vi "Test Compare Clusters.vi"(11 "Dummy In":refnum<class "Example Test Case.lvclass">) -> (0 "error out":errorcluster, 3 "Dummy Out":refnum<class "Example Test Case.lvclass">)   [LabVIEW 2020, in "Example Test Case.lvclass"]
doc: "Test case with comparison"
uses:
  Example Test Case.lvclass
  C:/git/astemes-lunit/source/LUnit Test Case.lvclass
  LUnit Test Case.lvclass/LUnit Test Case.ctl
  c67ca9b7-f05b-4050-9a64-1f171d30ec2c.vi
  Core/LUnit Test Case/Private/Append Pass Result.vi
  Core/LUnit Test Case/Private/Append Fail Result.vi
  c67ca9b7-f05b-4050-9a64-1f171d30ec2c.vi/9c5d11cd-9439-4240-a1ee-d9baace9c924.vi
  Core/LUnit Test Case/Private/Run In UI.vi
  <vilib>/Utility/error.llb/Clear Errors.vi
  Example Test Case.lvclass/Example Test Case.ctl
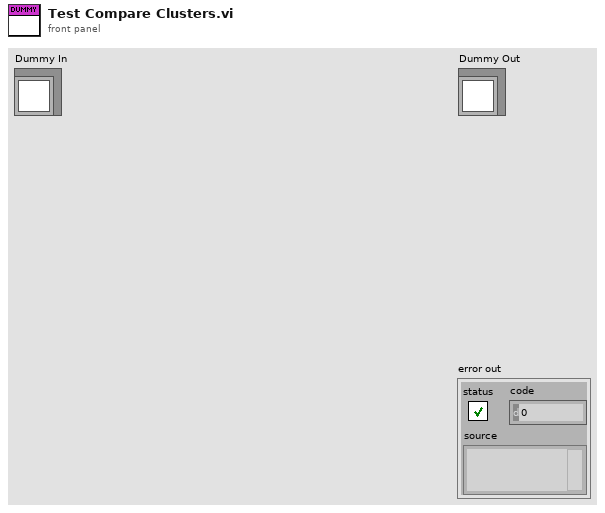
[diagram p1: front panel]
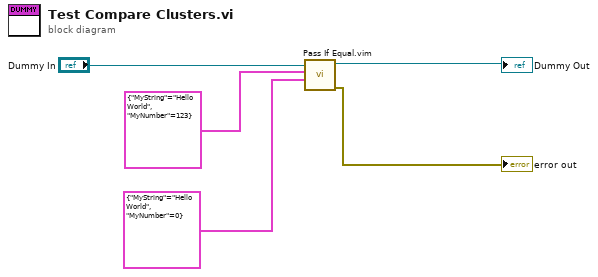
[diagram p0: block diagram]
diagram:
  n1 = call "Pass If Equal.vim"("Actual"=cluster{"MyString":string, "MyNumber":i32} {"MyString"="Hello World", "MyNumber"=0}, "Expected"=cluster{"MyString":string, "MyNumber":i32} {"MyString"="Hello World", "MyNumber"=123}, "LUnit Test Case In"="Dummy In") -> ("error out"=→"error out":errorcluster, "LUnit Test Case Out"=→"Dummy Out":refnum<class "Example Test Case.lvclass">)  [unwired: 7 in]
